vi "Select a new macro line.vi"(8 "error in (no error)":errorcluster, 9 "Index IN":i32, 10 "Clicked Table reference":refnum<vi>, 11 "UI control refnums":T1) -> (0 "error out":errorcluster, 2 "Index Out":i32)   [LabVIEW 2012]
doc: "SciScan 1.2 160622"
uses:
  Custom Controls and Typedefs/Macro_MD_UI Control Refnums.ctl
  Custom Controls and Typedefs/Delete Button.ctl
  Custom Controls and Typedefs/Edit Button.ctl
  Custom Controls and Typedefs/Timing Estimate Cluster.ctl
  CommonResource VIs/Timing/Timing Indicator.ctl
  Custom Controls and Typedefs/Load from PSM Button.ctl
  CommonResource VIs/FormatTree&TableStyle_Commands.ctl
panel:
  # "(hh:mm:ss)"
  # "(hh:mm:ss)"
  # "(hh:mm:ss)"
  # "(hh:mm:ss)"
  # "(hh:mm:ss)"
  # "(hh:mm:ss)"
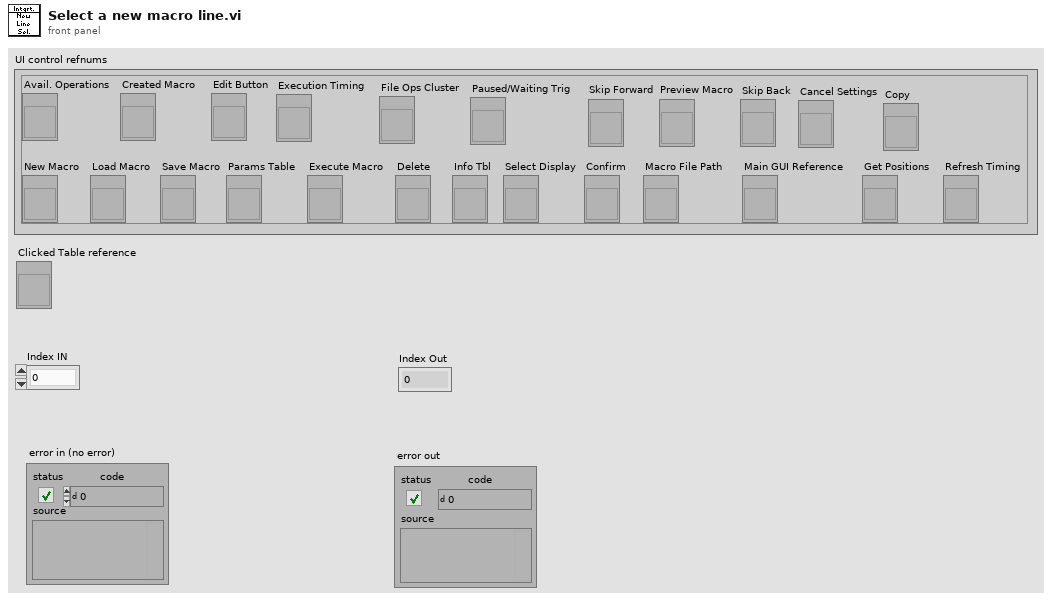
[diagram p1: front panel]
types:
  T1 = typedef "Macro_MD_UI Control Refnums.ctl" = cluster{"Avail. Operations":refnum<vi>, "Created Macro":refnum<vi>, "Load Macro":refnum<vi>, "Save Macro":refnum<vi>, "Params Table":refnum<vi>, "Delete":refnum<vi>, "Edit Button":refnum<vi>, "Execute Macro":refnum<vi>, "Info Tbl":refnum<vi>, "Execution Timing":refnum<vi>, "Select Display":refnum<vi>, "File Ops Cluster":refnum<vi>, "Paused/Waiting Trig":refnum<vi>, "Confirm":refnum<vi>, "New Macro":refnum<vi>, "Preview Macro":refnum<vi>, "Skip Forward":refnum<vi>, "Skip Back":refnum<vi>, "Macro File Path":refnum<vi>, "Main GUI Reference":refnum<vi>, "Cancel Settings":refnum<vi>, "Get Positions":refnum<vi>, "Copy":refnum<vi>, "Refresh Timing":refnum<vi>}
  T2 = typedef "LVRowAndColumnTypeDef.ctl" = cluster{"Row":i32, "Column":i32}
  T3 = typedef "FormatTree&TableStyle_Commands.ctl" = enum16{"Colour Row", "Uncolour Row", "Bold Row", "Unbold Row", "Clear", "UpdateVisibleRows"}
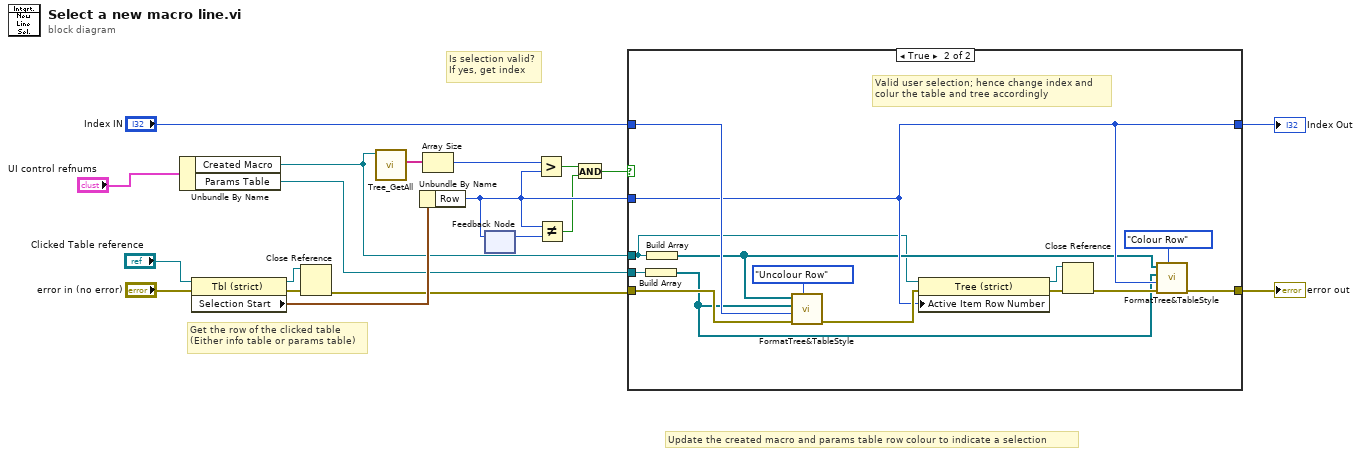
[diagram p0: block diagram]
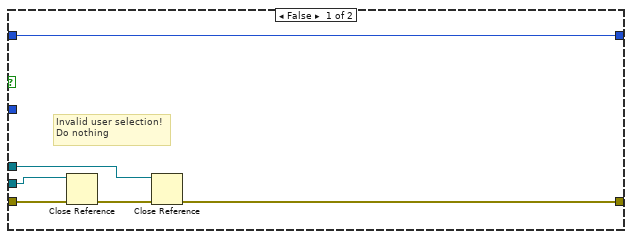
[diagram p2: hidden frame]
diagram:
  # "Update the created macro and params table row colour to indicate a selection"
  # "Get the row of the clicked table\n(Either info table or params table)"
  # "Is selection valid?\nIf yes, get index"
  n1 = Unbundle By Name("UI control refnums") -> ("Created Macro"=w5:refnum<vi>, "Params Table"=w1:refnum<vi>)
  n2 = property class="Tbl (strict)"(reference="Clicked Table reference", error in="error in (no error)") -> (reference out=w3:refnum<vi>, error out=w4:errorcluster, "Selection Start"=w16:T2)
  n3 = Close Reference(reference=w3, error in (no error)=w4) -> (error out=w2:errorcluster)
  n4 = call "Tree_GetAll.vi"("Tree Refnum IN"=w5) -> ("Tags"=w18:string[])  [unwired: 7 in, 3 out]
  n5 = Unbundle By Name(w16) -> ("Row"=w14:i32)
  n6 = Array Size(array=w18) -> (size(s)=w19:i32)
  n7 = feedback #1() -> (w17:i32)  [unwired: 1 in]
  n8 = feedback-in #1(w14) -> ()
  n9 = Greater?(x=w19, y=w14) -> (0:w15:bool)
  n10 = Not Equal?(x=w14, y=w17) -> (x != y?=w13:bool)
  n11 = And(x=w15, y=w13) -> (x .and. y?=w12:bool)
  n12 = case shown="True" w12 {
    tunnel: "Index IN" -> [w25 w35]
    tunnel: [w25 w32] -> w9
    tunnel: w1 -> [w21 w29]
    tunnel: w5 -> [w20 w26]
    tunnel: w14 -> [_ w32]
    tunnel: w2 -> [w24 w36]
    tunnel: [w22 w30] -> w8
    frame False {
      # "Invalid user selection!\nDo nothing"
      n13 = Close Reference(reference=w21, error in (no error)=w24) -> (error out=w23:errorcluster)
      n14 = Close Reference(reference=w20, error in (no error)=w23) -> (error out=w22:errorcluster)
    }
    frame True {
      # "Valid user selection; hence change index and\ncolur the table and tree accordingly"
      n15 = Build Array(w29) -> (w27:refnum<vi>[])
      n16 = Build Array(w26) -> (w28:refnum<vi>[])
      n17 = call "FormatTree&TableStyle.vi"("Format Command"=FormatTree&TableStyle_Commands."Uncolour Row", "Error In"=w36, "Row Index"=w35, "Array of Table references"=w27, "Array of Tree references"=w28) -> ("Error Out"=w34:errorcluster)  [unwired: 6 in]
      n18 = property class="Tree (strict)"(reference=w26, error in=w34, "Active Item Row Number"=w32) -> (reference out=w38:refnum<vi>, error out=w39:errorcluster)
      n19 = Close Reference(reference=w38, error in (no error)=w39) -> (error out=w31:errorcluster)
      n20 = call "FormatTree&TableStyle.vi"("Format Command"=FormatTree&TableStyle_Commands."Colour Row", "Error In"=w31, "Row Index"=w32, "Array of Table references"=w27, "Array of Tree references"=w28) -> ("Error Out"=w30:errorcluster)  [unwired: 6 in]
    }
  }
  "error out" <- w8
  "Index Out" <- w9
